vi "2d_InitSingle.vi"(8 "error in (no error)":errorcluster, 11 "MagSpecCamera in":refnum<class "MagSpecCamera.lvclass">) -> (0 "error out":errorcluster, 3 "MagSpecCamera in":refnum<class "MagSpecCamera.lvclass">)   [LabVIEW 2020, in "MagSpecCamera.lvclass"]
uses:
  MagSpecCamera.lvclass
  MagSpec_Bella/Controls/2D.ctl
  MagSpecCamera.lvclass/MagSpecCamera.ctl
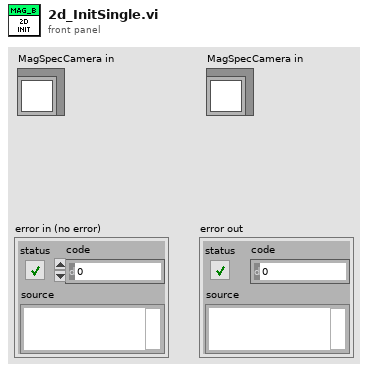
[diagram p1: front panel]
types:
  T1 = typedef "2D.ctl" = cluster{"dp":dbl[][], "chargeCompensation":dbl[][], "angle":dbl[][], "Momentum":dbl[][]}
  T2 = typedef "CameraSettings_File.ctl" = cluster{"FOV [mm]":dbl, "Left edge [mm]":dbl, "ROI Y offset":dbl, "ROI height":dbl, "ROI X offset":dbl, "ROI width":dbl, "Y center pixel":dbl, "Y Start":dbl, "Y End":dbl, "X Start":dbl, "X End":dbl, "rot [deg]":dbl}
  T3 = typedef "Calibration_Pixel_based.ctl" = cluster{"y1(pixel)":dbl[], "y2(pixel)":dbl[], "dp/B [MeV/C/B] (pixel)":dbl[], "energyDependence Input(pixel)":dbl[], "bending angle [deg](pixel)":dbl[], "total path(pixel)":dbl[], "pixel angle (y)(pixel)":dbl[], "energy dependence (pixel)":dbl[], "charge compensation (pixel)":dbl[], "Momentum [MeV/C](pixel)":dbl[], "angular compensation(pixel)":dbl[]}
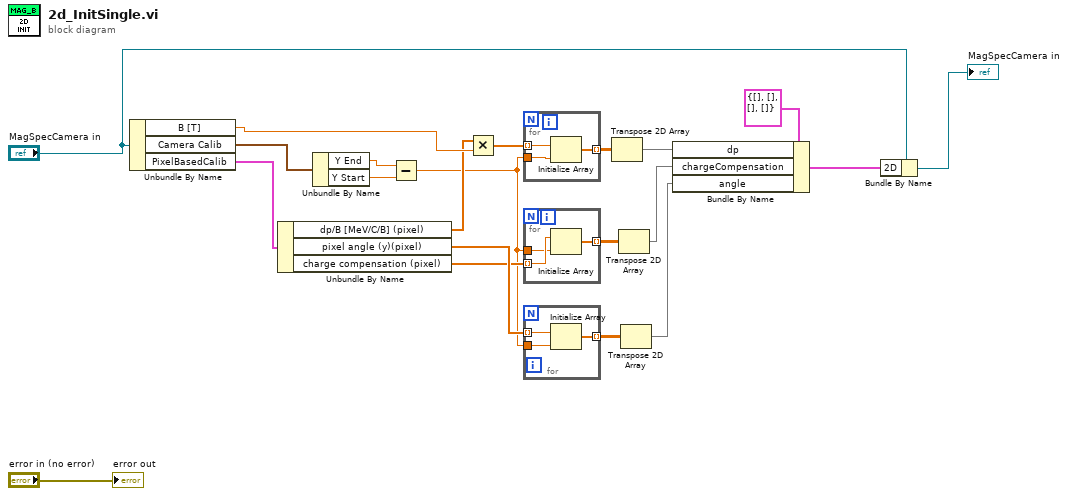
[diagram p0: block diagram]
diagram:
  n1 = Unbundle By Name("MagSpecCamera in") -> ("B [T]"=w16:dbl, "Camera Calib"=w18:T2, "PixelBasedCalib"=w19:T3)
  n2 = Unbundle By Name(w19) -> ("dp/B [MeV/C/B] (pixel)"=w6:dbl[], "pixel angle (y)(pixel)"=w10:dbl[], "charge compensation (pixel)"=w5:dbl[])
  n3 = Unbundle By Name(w18) -> ("Y End"=w3:dbl, "Y Start"=w1:dbl)
  n4 = Subtract(x=w3, y=w1) -> (x-y=w2:dbl)
  n5 = Multiply(x=w6, y=w16) -> (x*y=w12:dbl[])
  n6 = for {
    tunnel: w12 -> [w24] mode=indexing
    tunnel: [w23] -> w13 mode=indexing
    tunnel: w2 -> [w22]
    n7 = Initialize Array(w24, w22) -> (w23:dbl[])
  }
  n8 = for {
    tunnel: w5 -> [w27] mode=indexing
    tunnel: [w26] -> w11 mode=indexing
    tunnel: w2 -> [w25]
    n9 = Initialize Array(w27, w25) -> (w26:dbl[])
  }
  n10 = for {
    tunnel: w10 -> [w30] mode=indexing
    tunnel: [w29] -> w14 mode=indexing
    tunnel: w2 -> [w28]
    n11 = Initialize Array(w30, w28) -> (w29:dbl[])
  }
  n12 = Transpose 2D Array(2D array=w13) -> (transposed array=w9:dbl[][])
  n13 = Transpose 2D Array(2D array=w11) -> (transposed array=w7:dbl[][])
  n14 = Transpose 2D Array(2D array=w14) -> (transposed array=w8:dbl[][])
  n15 = Bundle By Name(cluster=T1 {"dp"=[], "chargeCompensation"=[], "angle"=[], "Momentum"=[]} ("2D"), "dp"=w9, "chargeCompensation"=w7, "angle"=w8) -> (w15:T1)
  n16 = Bundle By Name(cluster="MagSpecCamera in", "2D"=w15) -> (→"MagSpecCamera in":refnum<class "MagSpecCamera.lvclass">)
  "error out" <- "error in (no error)"
